vi "Generate Trace for New Actor.vi"(8 "Debug Alias":string, 9 "Class Name":string, 10 "Actor Enqueuer":refnum<class "Message Enqueuer.lvclass">, 11 "Caller Enqueuer":refnum<class "Message Enqueuer.lvclass">) -> ()   [LabVIEW 2025, in "Actor Framework.lvlib"]
doc: "Generates a DETT User Generated Trace for an actor being newly launched."
uses:
  Actor Framework.lvlib
  Message Enqueuer/Message Enqueuer.lvclass
  Support/Registration Mode.ctl
  Support/Localized Strings.vi
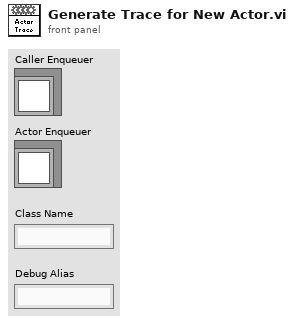
[diagram p1: front panel]
types:
  T1 = typedef "Actor Framework.lvlib/Registration Mode.ctl" = enum16{"Register Actor", "Get ID", "Get Enqueuer", "Deregister Actor", "Get Update Event", "Get All Actors", "Set Actor Core Name"}
  T2 = typedef "Actor Framework.lvlib/This Actor.ctl" = cluster{"Enqueuer":refnum<class "Message Enqueuer.lvclass">, "ID":string, "Alias":string, "Actor Core Name":string, "Details":cluster{"Qualified Name":string, "Caller ID":string}}
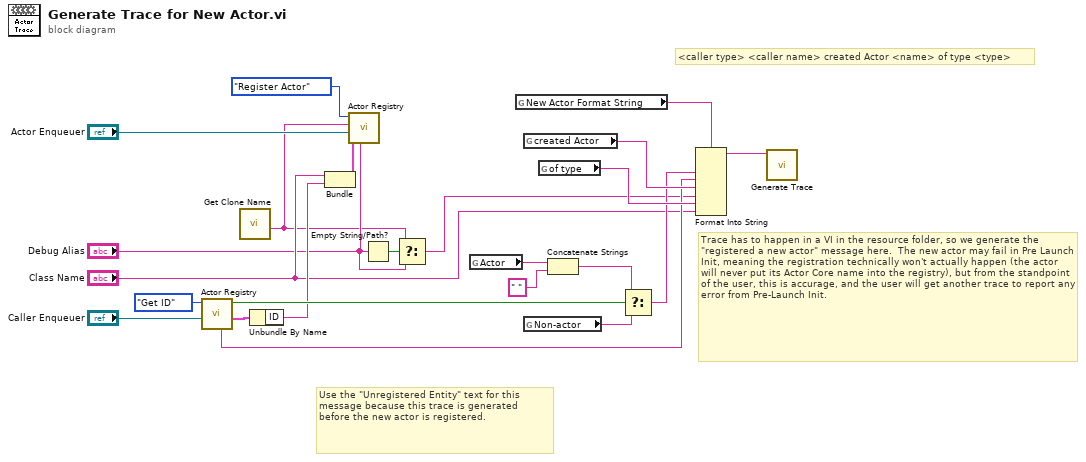
[diagram p0: block diagram]
diagram:
  # "Use the \"Unregistered Entity\" text for this message because this trace is generated before the new actor is registered."
  # "Trace has to happen in a VI in the resource folder, so we generate the \"registered a new actor\" message here.  The new actor may fail in Pre Launch Init, meaning the registration technically won't actually happen (the actor will never put its Actor Core name into the registry), but from the standpoint of the user, this is accurage, and the user will get another trace to report any error from Pre-Launch Init."
  # "<caller type> <caller name> created Actor <name> of type <type>"
  n1 = call "Actor Registry.vi"("Actor Enqueuer"="Caller Enqueuer", "Action"=Registration_Mode."Get ID") -> ("This Actor"=w23:T2, "Found"=w11:bool, "Actor Alias out"=w10:string)  [unwired: 5 in, 2 out]
  n2 = call "Get Clone Name.vi"() -> ("Clone ID"=w1:string)  [unwired: 10 in, 1 out]
  n3 = Unbundle By Name(w23) -> ("ID"=w9:string)
  n4 = Bundle("Class Name"="Class Name", "ID"=w9) -> (w4:cluster{"Class Name":string, "ID":string})  [unwired: 1 in]
  n5 = call "Actor Registry.vi"("Actor Alias"="Debug Alias", "Details"=w4, "Actor Enqueuer"="Actor Enqueuer", "Actor ID"=w1, "Action"=Registration_Mode."Register Actor") -> ()  [unwired: 2 in, 5 out]
  n6 = Empty String/Path?(string/path="Debug Alias") -> (empty?=w8:bool)
  n7 = Select(t=w1, s=w8, f="Debug Alias") -> (s? t:f=w6:string)
  n8 = global read "Localized Strings.vi" "Actor"() -> (w17:string)
  n9 = global read "Localized Strings.vi" "New Actor Format String"() -> (w13:string)
  n10 = global read "Localized Strings.vi" "created Actor"() -> (w14:string)
  n11 = global read "Localized Strings.vi" "Non-actor"() -> (w16:string)
  n12 = global read "Localized Strings.vi" "of type"() -> (w15:string)
  n13 = Concatenate Strings(w17, " " ("string")) -> (w18:string)
  n14 = Select(t=w18, s=w11, f=w16) -> (s? t:f=w12:string)
  n15 = Format Into String(format string=w13, w12, w10, w14, w6, w15, "Class Name") -> (resulting string=w20:string)  [unwired: 2 in, 1 out]
  n16 = call "Generate Trace.vi"("String"=w20) -> ()  [unwired: 11 in]
